vi "APTmotorSet.vi"(8 "error in (no error)":errorcluster, 10 "Set position":sgl[](array[numeric]) min=0 max=500, 11 "reference in":refnum<k7>[](array[refnum])) -> (0 "error out":errorcluster, 3 "reference out":refnum<k7>[](array[refnum]))   [LabVIEW 2013]
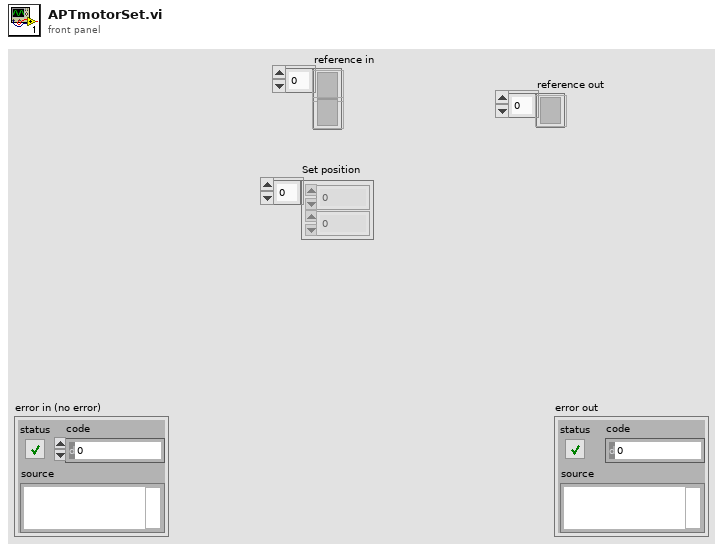
[diagram p1: front panel]
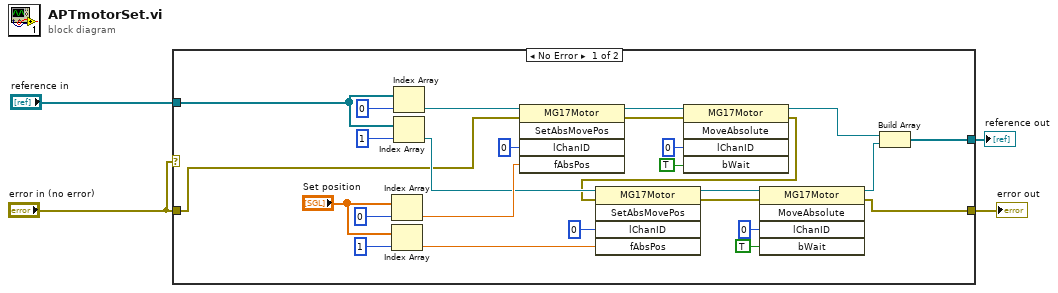
[diagram p0: block diagram]
diagram:
  n1 = case shown="No Error" "error in (no error)" {
    tunnel: [w5 w32] -> w4
    tunnel: "error in (no error)" -> [w15 w32]
    tunnel: [w10 w31] -> w2
    tunnel: "reference in" -> [w9 w31]
    frame No Error {
      n2 = Index Array(array="Set position", index=0) -> (element=w21:sgl)
      n3 = Index Array(array="Set position", index=1) -> (element=w17:sgl)
      n4 = Index Array(array=w9, index=0) -> (element=w29:refnum<k7>)
      n5 = Index Array(array=w9, index=1) -> (element=w18:refnum<k7>)
      n6 = invoke class="MG17Motor" method="SetAbsMovePos"(reference=w29, error in=w15, "lChanID"=0, "fAbsPos"=w21) -> (reference out=w26:refnum<k7>, error out=w13:errorcluster)  [unwired: 1 in, 3 out]
      n7 = invoke class="MG17Motor" method="MoveAbsolute"(reference=w26, error in=w13, "lChanID"=0, "bWait"=TRUE) -> (reference out=w12:refnum<k7>, error out=w6:errorcluster)  [unwired: 1 in, 3 out]
      n8 = invoke class="MG17Motor" method="SetAbsMovePos"(reference=w18, error in=w6, "lChanID"=0, "fAbsPos"=w17) -> (reference out=w19:refnum<k7>, error out=w14:errorcluster)  [unwired: 1 in, 3 out]
      n9 = invoke class="MG17Motor" method="MoveAbsolute"(reference=w19, error in=w14, "lChanID"=0, "bWait"=TRUE) -> (reference out=w11:refnum<k7>, error out=w5:errorcluster)  [unwired: 1 in, 3 out]
      n10 = Build Array(w12, w11) -> (w10:refnum<k7>[])
    }
    frame Error {
    }
  }
  "error out" <- w4
  "reference out" <- w2
